vi "Modbus Check Sequence Status.vi"(11 "Input Registers":u16[](array[numeric])) -> (2 "Test chamber is in sequence - LDO":bool, 3 "Test chamber is in sequence - FVIR":bool)   [LabVIEW 2023, in "Modbus.lvlib"]
uses:
  Modbus.lvlib
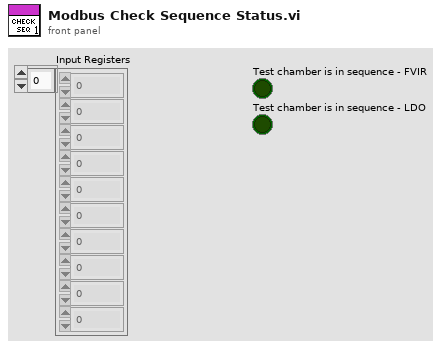
[diagram p1: front panel]
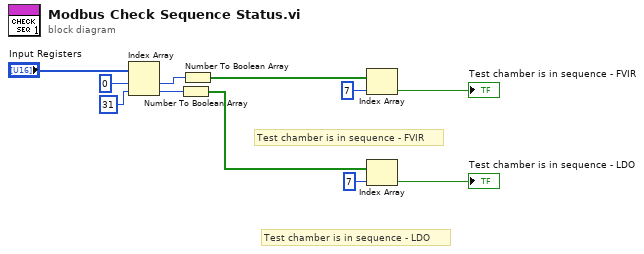
[diagram p0: block diagram]
diagram:
  # "Test chamber is in sequence - LDO"
  # "Test chamber is in sequence - FVIR"
  n1 = Index Array(array="Input Registers", index #1=0 ("index"), index #2=31 ("index")) -> (element #1=w4:u16, element #2=w9:u16)
  n2 = Number To Boolean Array(number=w9) -> (Boolean array=w11:bool[])
  n3 = Number To Boolean Array(number=w4) -> (Boolean array=w6:bool[])
  n4 = Index Array(array=w6, index=7) -> (element=→"Test chamber is in sequence - FVIR":bool)
  n5 = Index Array(array=w11, index=7) -> (element=→"Test chamber is in sequence - LDO":bool)
